vi "Noise-Globals.vi"() -> ()   [LabVIEW 2020]
uses:
  4th Generation/Classes/Filter/Filter.lvclass
panel:
  in  "Filter":refnum<class "Filter.lvclass">
  in  "Noise.Vrms":dbl=0.25
  out "Gaussian":bool=TRUE
  in  "Noise":dbl[](array[numeric])
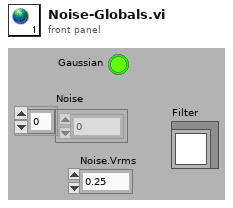
[diagram p1: front panel]
diagram:
